vi "QFontDialog.vi"(5 "parent":refnum<class "QWidget.lvclass">, 8 "Error In":errorcluster, 10 "initial":refnum<class "QFont.lvclass">, 11 "Post-Bundled Subclass":refnum<class "QFontDialog.lvclass">) -> (0 "Error Out":errorcluster, 3 "New QFontDialog":refnum<class "QFontDialog.lvclass">)   [LabVIEW 2014, in "QFontDialog.lvclass"]
doc: "LabVIEW-specific documentation is not yet available. See <b>https://doc.qt.io/qt-5/qfontdialog.html#QFontDialog</b>"
uses:
  QFontDialog.lvclass
  Qt GUI/QFont/QFont.lvclass
  QWidget/QWidget.lvclass
  LQ Core/LQCoreEngine/_Internal/LQIdentity Registry Action.ctl
  LQ Core/LQSerialData/LQSerialData.lvclass/LQSerialData.ctl
  LQ Core/LQIdentity/LQIdentity.lvclass/LQIdentity.ctl
  LQ Core/LQCoreEngine/LQCoreEngine.lvclass
  LQ Core/LQ Core.lvlib
  LQ Core/LQIdentity/LQIdentity.lvclass
  LQ Core/LQSerialData/LQSerialData.lvclass
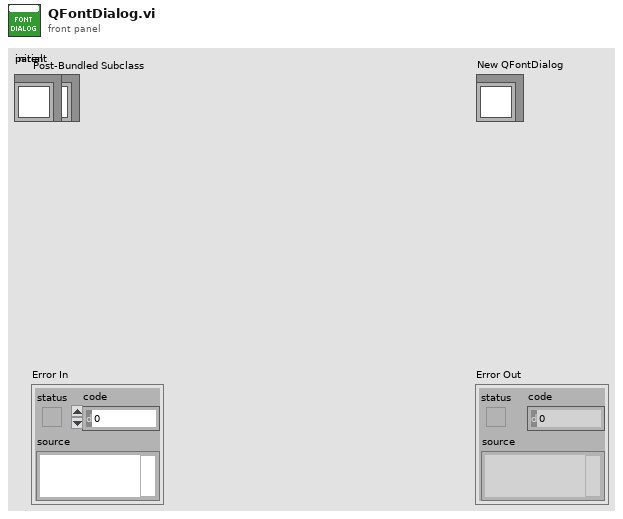
[diagram p1: front panel]
types:
  T1 = typedef "LQ Core.lvlib/LQCoreEngine.lvclass/LQIdentity Registry Action.ctl" = enum16{"Init", "Register LQIdentity", "Get LQIdentity Info", "Deregister LQIdentity"}
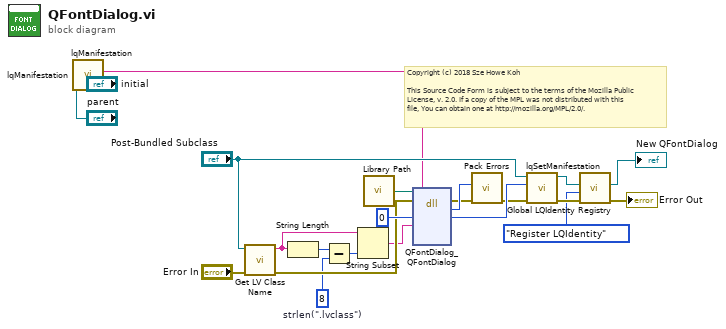
[diagram p0: block diagram]
diagram:
  w8 = 8  # strlen(".lvclass")
  # "Copyright (c) 2018 Sze Howe Koh\n\nThis Source Code Form is subject to the terms of the Mozilla Public\nLicense, v. 2.0. If a copy of the MPL was not distributed with this\nfile, You can obtain one at http://mozilla.org/MPL/2.0/."
  n1 = call "lqManifestation.vi"("LQIdentity in"="parent") -> ("Manifestation"=w1:u64)  [unwired: 9 in, 1 out]
  n2 = call "lqManifestation.vi"("LQSerialData in"="initial") -> ("Manifestation"=w3:string)  [unwired: 9 in, 1 out]
  n3 = call <vilib>:"Get LV Class Name.vi"("error in (no error)"="Error In", "object"="Post-Bundled Subclass") -> ("error out"=w10:errorcluster, "class name"=w6:string)  [unwired: 8 in]
  n4 = String Length(string=w6) -> (length=w9:i32)
  n5 = Subtract(x=w9, y=w8) -> (x-y=w7:i32)
  n6 = String Subset(string=w6, length (rest)=w7) -> (substring=w5:string)  [unwired: 1 in]
  n7 = call "Library Path.vi"() -> ("Library Path"=w21:path)
  n8 = dll-call lib="?" fn="QFontDialog_QFontDialog"(path in=w21, error in=w10, "_retVal"=u64 0 ("_instance"), "_className"=w5, "initial"=w3, "parent"=w1) -> (error out=w19:errorcluster, w20:i32, "_retVal"=w22:u64)  [unwired: 4 in, 1 out]
  n9 = call "Pack Errors.vi"("Error In"=w19, "Error Code"=w20) -> ("Error Out"=w18:errorcluster)  [unwired: 9 in]
  n10 = call "lqSetManifestation.vi"("Error In"=w18, "Manifestation"=w22, "LQIdentity in"="Post-Bundled Subclass") -> ("Error Out"=w16:errorcluster, "LQIdentity out"=w17:refnum<class "QFontDialog.lvclass">)  [unwired: 7 in]
  n11 = call "Global LQIdentity Registry.vi"("Error In"=w16, "Registry Action"=LQIdentity_Registry_Action."Register LQIdentity", "LQIdentity Info In"=w17) -> ("Error Out"=→"Error Out":errorcluster, "LQIdentity Info Out"=→"New QFontDialog":refnum<class "QFontDialog.lvclass">)  [unwired: 7 in]
